vi "NeighbourProximity.vi"(6 "MaxInterval":dbl, 7 "Values":dbl[](array[numeric]), 11 "InterpolatedIndex":dbl) -> (1 "useInterpolated":bool, 3 "IndexToUse":dbl)   [LabVIEW 2020]
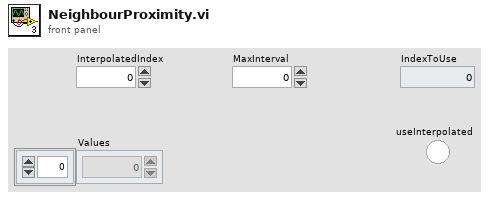
[diagram p1: front panel]
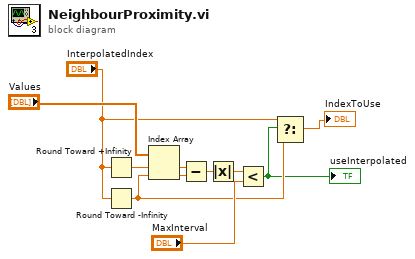
[diagram p0: block diagram]
diagram:
  n1 = Round Toward +Infinity(x="InterpolatedIndex") -> (ceil(x): smallest int >= x=w2:dbl)
  n2 = Round Toward -Infinity(1:"InterpolatedIndex") -> (0:w8:dbl)
  n3 = Index Array(array="Values", index #1=w2, index #2=w8) -> (element #1=w3:dbl, element #2=w4:dbl)
  n4 = Subtract(x=w3, y=w4) -> (x-y=w5:dbl)
  n5 = Absolute Value(x=w5) -> (abs(x)=w11:dbl)
  n6 = Less?(x=w11, y="MaxInterval") -> (x < y?=w7:bool)
  "useInterpolated" <- w7
  n7 = Select(t="InterpolatedIndex", s=w7, f=w8) -> (s? t:f=→"IndexToUse":dbl)
